vi "Grab Weight.vi"(8 "error in":errorcluster, 10 "Weight Number":i32, 11 "GrabberTool in":refnum<class "GrabberTool Class.lvclass">) -> (0 "error out":errorcluster, 3 "GrabberTool out":refnum<class "GrabberTool Class.lvclass">)   [LabVIEW 2011, in "GrabberTool Class.lvclass"]
uses:
  GrabberTool Class.lvclass
  Config Manager Class/Type Definitions/Part Type.ctl
  Config Manager Class/Type Definitions/Offset.ctl
  Config Manager Class/Type Definitions/Named Position.ctl
  WorkTable Class/WorkTable Class.lvclass
  Vec3d Class/Vec3d Class.lvclass
  Config Manager Class/Read Geometry Definition 3D.vi
  Config Manager Class/Config Manager Class.lvclass
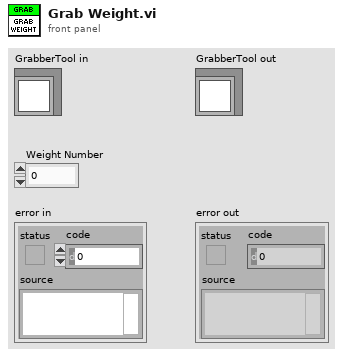
[diagram p1: front panel]
types:
  T1 = typedef "Part Type.ctl" = enum16{"BBM", "HDI", "BARE HDI", "GLUERESERVOIR", "STAMP_1", "STAMP_2", "STAMP_3", "STAMP_4", "STAMP_5", "WEIGHT_1", "WEIGHT_2", "WEIGHT_3", "WEIGHT_4", "WEIGHT_5", "WEIGHT_6", "WEIGHT_7", "WEIGHT_8", "PICKER_TOOL", "GRABER_TOOL"}
  T2 = typedef "Offset.ctl" = enum16{"needle_offset", "tool_holder_offset"}
  T3 = typedef "Named Position.ctl" = enum16{"home", "module_chuck_0", "module_chuck_1", "module_chuck_2", "module_chuck_3", "module_chuck_4", "glue_reservoir_chuck", "stamp_tool_chuck", "weight_tool_chuck", "needle_calibration", "tool_rack_pos_0_in", "tool_rack_pos_0_out", "tool_rack_pos_1_in", "tool_rack_pos_1_out", "tool_rack_pos_2_in", "tool_rack_pos_2_out", "front_load_position", "grabber_start_pos"}
  T4 = typedef "Worktable_Weights.ctl" = cluster{"Weight Slots":cluster{"Weight State":enum16{"Empty", "Populated"}, "Weight Type":enum16{"Weight 1", "Weight 2", "Weight 3", "Weight 4"}, "Location/Orientation":T5}[], "Vacuum Channel":i32}
  T5 = typedef "Position_Orientation.ctl" = cluster{"Center":refnum<class "Vec3d Class.lvclass">, "Orientation":refnum<class "Orient3d Class.lvclass">}
  T6 = cluster{"Weight State":enum16{"Empty", "Populated"}, "Weight Type":enum16{"Weight 1", "Weight 2", "Weight 3", "Weight 4"}, "Location/Orientation":T5}[]
  T7 = cluster{"Weight State":enum16{"Empty", "Populated"}, "Weight Type":enum16{"Weight 1", "Weight 2", "Weight 3", "Weight 4"}, "Location/Orientation":T5}
  T8 = typedef "Gluing Parameters.ctl" = cluster{"Safe Grabber Pickup":dbl, "Safe Grabber Lift":dbl}
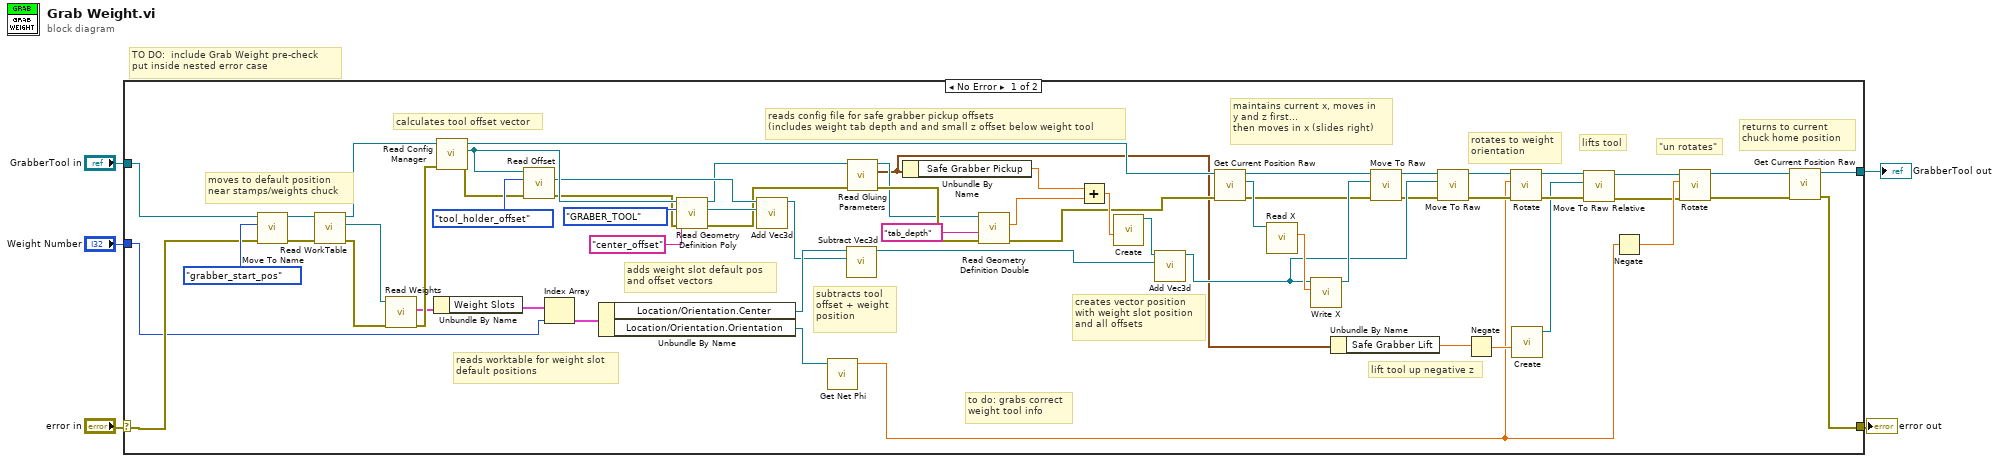
[diagram p0: block diagram]
diagram:
  # "TO DO:  include Grab Weight pre-check\nput inside nested error case"
  n1 = case shown="No Error" "error in" {
    selector: "error in" -> [w60 w66]
    tunnel: [w6 w66] -> w4
    tunnel: [w7 w65] -> w2
    tunnel: "GrabberTool in" -> [w63 w65]
    tunnel: "Weight Number" -> [w37 _]
    frame No Error {
      # "lift tool up negative z"
      # "to do: grabs correct\nweight tool info"
      # "subtracts tool\noffset + weight\nposition"
      # "returns to current \nchuck home position"
      # "\"un rotates\""
      # "lifts tool"
      # "rotates to weight\norientation"
      # "maintains current x, moves in \ny and z first...\nthen moves in x (slides right)"
      # "creates vector position\nwith weight slot position\nand all offsets"
      # "reads config file for safe grabber pickup offsets\n(includes weight tab depth and and small z offset below weight tool"
      # "adds weight slot default pos\nand offset vectors"
      # "reads worktable for weight slot\ndefault positions"
      # "calculates tool offset vector"
      # "moves to default position\nnear stamps/weights chuck"
      n2 = call-dynamic "Move To Name.vi"("error in"=w60, "Destination"=Named_Position."grabber_start_pos", "Gantry in"=w63) -> ("error out"=w59:errorcluster, "Gantry out"=w62:refnum<class "GrabberTool Class.lvclass">)  [unwired: 7 in]
      n3 = call-dynamic "Read WorkTable.vi"("error in"=w59, "Gantry Class in"=w62) -> ("error out"=w58:errorcluster, "WorkTable Class.lvclass"=w56:refnum<class "WorkTable Class.lvclass">, "Gantry Class out"=w61:refnum<class "GrabberTool Class.lvclass">)  [unwired: 7 in]
      n4 = call-dynamic "Read Weights.vi"("error in (no error)"=w58, "WorkTable Class in"=w56) -> ("error out"=w57:errorcluster, "Weights"=w55:T4)  [unwired: 7 in, 1 out]
      n5 = Unbundle By Name(w55) -> ("Weight Slots"=w54:T6)
      n6 = call-dynamic "Read Config Manager.vi"("error in"=w57, "Gantry in"=w61) -> ("error out"=w43:errorcluster, "Config Manager"=w51:refnum<class "Config Manager Class.lvclass">, "Gantry out"=w31:refnum<class "GrabberTool Class.lvclass">)  [unwired: 7 in]
      n7 = call "Read Offset.vi"("error in"=w43, "Offset"=Offset."tool_holder_offset", "Config Manager in"=w51) -> ("error out"=w42:errorcluster, "Vec3d out"=w48:refnum<class "Vec3d Class.lvclass">)  [unwired: 6 in, 1 out]
      n8 = Index Array(array=w54, index=w37) -> (element=w53:T7)
      n9 = Unbundle By Name(w53) -> ("Location/Orientation.Center"=w46:refnum<class "Vec3d Class.lvclass">, "Location/Orientation.Orientation"=w44:refnum<class "Orient3d Class.lvclass">)
      n10 = call-poly "Read Geometry Definition Poly.vi"("error in"=w42, "Feature"="center_offset", "Part Type"=Part_Type."GRABER_TOOL", "Config Manager in"=w51) -> ("error out"=w41:errorcluster, "Feature Coordinates"=w47:refnum<class "Vec3d Class.lvclass">, "Config Manager out"=w39:refnum<class "Config Manager Class.lvclass">)  [unwired: 5 in]
      n11 = call-dynamic "Add Vec3d.vi"(10:"Vec3d Class in"=w47, 11:"Vec3d Class in"=w48) -> ("Vec3d Class out"=w45:refnum<class "Vec3d Class.lvclass">)  [unwired: 8 in, 1 out]
      n12 = call "Get Net Phi.vi"("Orient3d"=w44) -> ("phi(deg)"=w13:dbl)  [unwired: 8 in, 2 out]
      n13 = call "Subtract Vec3d.vi"("Vec3d in 2"=w45, "Vec3d in 1"=w46) -> ("Vec3d Class out"=w32:refnum<class "Vec3d Class.lvclass">)  [unwired: 8 in, 1 out]
      n14 = call "Read Gluing Parameters.vi"("error in (no error)"=w41, "Config Manager Class in"=w39) -> ("error out"=w40:errorcluster, "Gluing Parameters"=w19:T8)  [unwired: 7 in, 1 out]
      n15 = Unbundle By Name(w19) -> ("Safe Grabber Pickup"=w35:dbl)
      n16 = call "Read Geometry Definition Double.vi"("error in"=w40, "Feature"="tab_depth", "Config Manager in"=w39) -> ("error out"=w23:errorcluster, "Geometry Definition"=w36:dbl)  [unwired: 6 in, 1 out]
      n17 = Add(x=w35, y=w36) -> (x+y=w34:dbl)
      n18 = call "Create.vi"("Z"=w34) -> ("Vec3d Class out"=w33:refnum<class "Vec3d Class.lvclass">)  [unwired: 9 in, 1 out]
      n19 = call-dynamic "Add Vec3d.vi"(10:"Vec3d Class in"=w32, 11:"Vec3d Class in"=w33) -> ("Vec3d Class out"=w24:refnum<class "Vec3d Class.lvclass">)  [unwired: 8 in, 1 out]
      n20 = call-dynamic "Get Current Position Raw.vi"("error in"=w23, "Gantry in"=w31) -> ("error out"=w22:errorcluster, "Vec3d Class out"=w27:refnum<class "Vec3d Class.lvclass">, "Gantry out"=w30:refnum<class "GrabberTool Class.lvclass">)  [unwired: 7 in]
      n21 = call-dynamic "Read X.vi"("Vec3d Class in"=w27) -> ("X"=w26:dbl)  [unwired: 8 in, 2 out]
      n22 = call-dynamic "Write X.vi"("X"=w26, "Vec3d Class in"=w24) -> ("Vec3d Class out"=w25:refnum<class "Vec3d Class.lvclass">)  [unwired: 8 in, 1 out]
      n23 = Unbundle By Name(w19) -> ("Safe Grabber Lift"=w18:dbl)
      n24 = call-dynamic "Move To Raw.vi"("error in"=w22, "Destination"=w25, "Gantry in"=w30) -> ("error out"=w21:errorcluster, "Gantry out"=w29:refnum<class "GrabberTool Class.lvclass">)  [unwired: 7 in]
      n25 = call-dynamic "Move To Raw.vi"("error in"=w21, "Destination"=w24, "Gantry in"=w29) -> ("error out"=w20:errorcluster, "Gantry out"=w28:refnum<class "GrabberTool Class.lvclass">)  [unwired: 7 in]
      n26 = Negate(x=w18) -> (-x=w17:dbl)
      n27 = call-dynamic "Rotate.vi"("error in"=w20, "distance(deg)"=w13, "Gantry in"=w28) -> ("error out"=w15:errorcluster, "Gantry out"=w16:refnum<class "GrabberTool Class.lvclass">)  [unwired: 7 in]
      n28 = call "Create.vi"("Z"=w17) -> ("Vec3d Class out"=w14:refnum<class "Vec3d Class.lvclass">)  [unwired: 9 in, 1 out]
      n29 = call-dynamic "Move To Raw Relative.vi"("error in"=w15, "Delta"=w14, "Gantry in"=w16) -> ("error out"=w10:errorcluster, "Gantry out"=w11:refnum<class "GrabberTool Class.lvclass">)  [unwired: 7 in]
      n30 = Negate(x=w13) -> (-x=w12:dbl)
      n31 = call-dynamic "Rotate.vi"("error in"=w10, "distance(deg)"=w12, "Gantry in"=w11) -> ("error out"=w8:errorcluster, "Gantry out"=w9:refnum<class "GrabberTool Class.lvclass">)  [unwired: 7 in]
      n32 = call-dynamic "Get Current Position Raw.vi"("error in"=w8, "Gantry in"=w9) -> ("error out"=w6:errorcluster, "Gantry out"=w7:refnum<class "GrabberTool Class.lvclass">)  [unwired: 7 in, 1 out]
    }
    frame Error {
    }
  }
  "error out" <- w4
  "GrabberTool out" <- w2
